vi "SVA 4MV6 T022 CCE.vi"(11 "SP":dbl(slide) scale=0.0..360.0) -> (3 "Posicion":cluster{dbl, dbl}(knob)={0.0, 349.0774854239136})   [LabVIEW 2020]
doc: "Ceballos Conde Emanuel 4MV6 Sistemas de visión artificial 2022/1\nEste VI realiza el control difuso de un SISTEMA SISO representado por un motor,el sisita tiene como entrada tiene la posición deseada y como salida un indicador de dos agujas donde la azul representa el valor solicitado y la roja el valor real"
uses:
  <vilib>/addons/Fuzzy Logic/TypeDefs/FL Defuzzification.ctl
  <vilib>/addons/Fuzzy Logic/TypeDefs/FL Antecedent Connective.ctl
  <vilib>/addons/Fuzzy Logic/TypeDefs/FL Consequent Implication.ctl
  <vilib>/addons/Fuzzy Logic/TypeDefs/FL Modifier.ctl
  <vilib>/addons/Fuzzy Logic/Membership/FL Create Membership Function (Triangle).vi
  <vilib>/addons/Fuzzy Logic/Membership/FL Create Membership Function (Trapezoid).vi
  <vilib>/addons/Fuzzy Logic/FL Fuzzy Controller (SISO).vi
  <vilib>/addons/Fuzzy Logic/NI_Fuzzy_Logic_API.lvlib
panel:
  in  "stop":bool
  # "Ceballos Conde Emanuel\n4MV6\nSistemas de visión artificial\n2022/1"
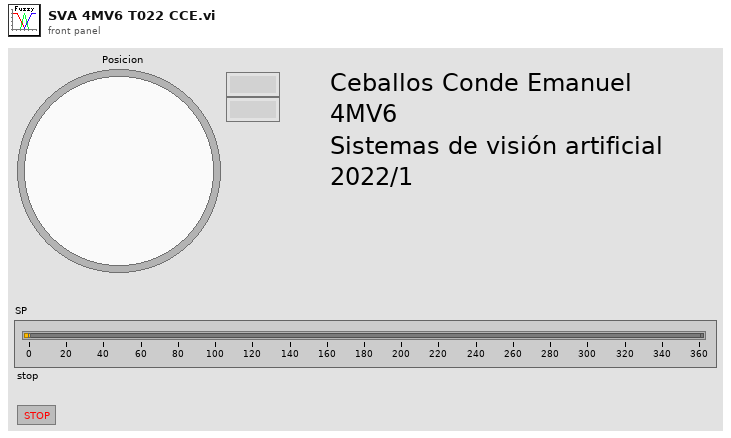
[diagram p1: front panel]
types:
  T1 = typedef "NI_Fuzzy_Logic_API.lvlib/FL Defuzzification.ctl" = u16
  T2 = typedef "NI_Fuzzy_Logic_API.lvlib/FL Membership Function.ctl" = cluster{"name":string, "shape":T3, "points":dbl[], "color":u32, "user-defined shape index":i32}
  T3 = typedef "NI_Fuzzy_Logic_API.lvlib/FL Membership Function Shape.ctl" = u16
  T4 = typedef "NI_Fuzzy_Logic_API.lvlib/FL Modifier.ctl" = u16
  T5 = typedef "NI_Fuzzy_Logic_API.lvlib/FL Consequent Implication.ctl" = u16
  T6 = typedef "NI_Fuzzy_Logic_API.lvlib/FL Antecedent Connective.ctl" = u16
  T7 = typedef "NI_Fuzzy_Logic_API.lvlib/FL Antecedent.ctl" = cluster{"Var Index":i32, "MF Index":i32, "Cond":T4}
  T8 = typedef "NI_Fuzzy_Logic_API.lvlib/FL Consequent.ctl" = cluster{"Var Index":i32, "MF Index":i32, "Cond":T4}
  T9 = typedef "NI_Fuzzy_Logic_API.lvlib/FL Rule.ctl" = cluster{"antecedents":T7[], "antecedent connective":T6, "consequents":T8[], "consequent implication":T5, "degree of support":dbl}
  T10 = typedef "NI_Fuzzy_Logic_API.lvlib/FL Variable.ctl" = cluster{"name":string, "range":dbl[], "MFs":T2[]}
  T11 = typedef "NI_Fuzzy_Logic_API.lvlib/FL System.ctl" = cluster{"input variables":T10[], "output variables":T10[], "rules":T9[], "defuzzification method":T1, "description":string, "user MF interpolating polynomials":T12[]}
  T12 = typedef "NI_Fuzzy_Logic_API.lvlib/FL Interpolating polynomials.ctl" = cluster{"X":dbl[], "Y":dbl[], "Y(x) coeff":dbl[][], "X(y) coeff":dbl[][], "Area(y) coeff":dbl[][], "coa_x(y) coeff":dbl[][]}
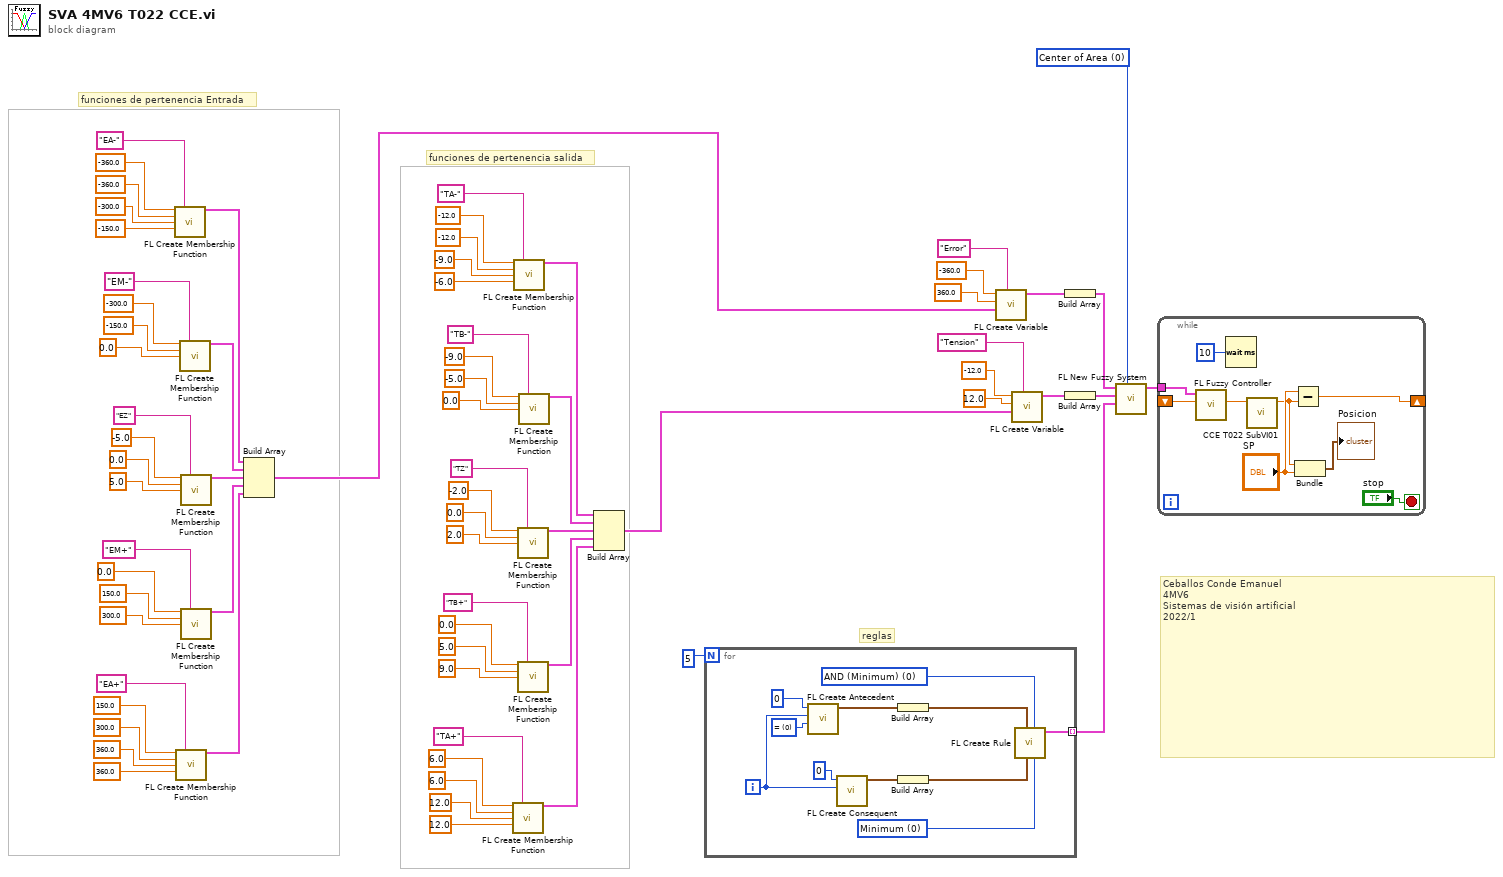
[diagram p0: block diagram]
diagram:
  w4 = T1 0 items=["Center of Area", "Modified Center of Area", "Center of Sums", "Center of Maximum", "Mean of Maximum"] ("defuzzification method")
  # "reglas"
  # "funciones de pertenencia salida"
  # "funciones de pertenencia Entrada"
  # "Ceballos Conde Emanuel\n4MV6\nSistemas de visión artificial\n2022/1"
  n1 = call-poly <vilib>:"FL Create Membership Function.vi"("left base"=-360.0, "name"="EA-", "left top"=-360.0 ("top"), "right top"=-300.0 ("right base"), "right base"=-150.0) -> ("membership function"=w63:T2)  [unwired: 9 in, 1 out]
  n2 = call-poly <vilib>:"FL Create Membership Function.vi"("left base"=150.0, "name"="EA+", "left top"=300.0 ("top"), "right top"=360.0 ("right base"), "right base"=360.0) -> ("membership function"=w42:T2)  [unwired: 9 in, 1 out]
  n3 = call-poly <vilib>:"FL Create Membership Function.vi"("left base"=-300.0, "name"="EM-", "top"=-150.0, "right base"=0.0) -> ("membership function"=w57:T2)  [unwired: 10 in, 1 out]
  n4 = call-poly <vilib>:"FL Create Membership Function.vi"("left base"=-5.0, "name"="EZ", "top"=0.0, "right base"=5.0) -> ("membership function"=w52:T2)  [unwired: 10 in, 1 out]
  n5 = call-poly <vilib>:"FL Create Membership Function.vi"("left base"=0.0, "name"="EM+", "top"=150.0, "right base"=300.0) -> ("membership function"=w47:T2)  [unwired: 10 in, 1 out]
  n6 = Build Array(w63, w57, w52, w47, w42) -> (w62:T2[])
  n7 = call-poly <vilib>:"FL Create Membership Function.vi"("left base"=6.0, "name"="TA+", "left top"=6.0 ("top"), "right top"=12.0 ("right base"), "right base"=12.0) -> ("membership function"=w9:T2)  [unwired: 9 in, 1 out]
  n8 = call-poly <vilib>:"FL Create Membership Function.vi"("left base"=-12.0, "name"="TA-", "left top"=-12.0 ("top"), "right top"=-9.0 ("right base"), "right base"=-6.0) -> ("membership function"=w30:T2)  [unwired: 9 in, 1 out]
  n9 = call-poly <vilib>:"FL Create Membership Function.vi"("left base"=-2.0, "name"="TZ", "top"=0.0, "right base"=2.0) -> ("membership function"=w19:T2)  [unwired: 10 in, 1 out]
  n10 = call-poly <vilib>:"FL Create Membership Function.vi"("left base"=0.0, "name"="TB+", "top"=5.0, "right base"=9.0) -> ("membership function"=w14:T2)  [unwired: 10 in, 1 out]
  n11 = call-poly <vilib>:"FL Create Membership Function.vi"("left base"=-9.0, "name"="TB-", "top"=-5.0, "right base"=0.0) -> ("membership function"=w24:T2)  [unwired: 10 in, 1 out]
  n12 = Build Array(w30, w24, w19, w14, w9) -> (w29:T2[])
  n13 = for {
    N: 5 -> [_]
    tunnel: [w71] -> w2 mode=indexing
    i -> [w74]
    w77 = T4 0 items=["=", "!="] ("condition")
    w80 = T5 0 items=["Minimum", "Product"] ("consequent implication")
    w81 = T6 0 items=["AND (Minimum)", "AND (Product)", "OR (Maximum)", "OR (Probabilistic)"] ("antecedent connective")
    n14 = call <vilib>:"FL Create Antecedent.vi"("condition"=w77, "membership function index"=w74, "variable index"=0) -> ("antecedent"=w79:T7)  [unwired: 7 in, 1 out]
    n15 = call <vilib>:"FL Create Consequent.vi"("membership function index"=w74, "variable index"=0) -> ("consequent"=w78:T8)  [unwired: 8 in, 1 out]
    n16 = Build Array(w79) -> (w73:T7[])
    n17 = Build Array(w78) -> (w72:T8[])
    n18 = call <vilib>:"FL Create Rule.vi"("consequent implication"=w80, "antecedent connective"=w81, "consequents"=w72, "antecedents"=w73) -> ("rule"=w71:T9)  [unwired: 6 in, 1 out]
  }
  n19 = call <vilib>:"FL Create Variable.vi"("name"="Error", "membership functions"=w62, "maximum"=360.0, "minimum"=-360.0) -> ("variable"=w40:T10)  [unwired: 6 in, 1 out]
  n20 = call <vilib>:"FL Create Variable.vi"("name"="Tension", "membership functions"=w29, "maximum"=12.0, "minimum"=-12.0) -> ("variable"=w7:T10)  [unwired: 6 in, 1 out]
  n21 = Build Array(w40) -> (w39:T10[])
  n22 = Build Array(w7) -> (w5:T10[])
  n23 = call <vilib>:"FL New Fuzzy System.vi"("defuzzification method"=w4, "rules"=w2, "output variables"=w5, "input variables"=w39) -> ("fuzzy system out"=w1:T11)  [unwired: 6 in, 1 out]
  n24 = while {
    shift-right: [w88] -> _
    shift-left: _ -> [w86]
    tunnel: w1 -> [w87]
    stop <- "stop" stop-if-true
    n25 = call-poly <vilib>:"FL Fuzzy Controller.vi"("input value"=w86, "fuzzy system in"=w87) -> ("output value"=w85:dbl)  [unwired: 5 in, 4 out]
    n26 = Wait (ms)(milliseconds to wait=u32 10) -> ()  [unwired: 1 out]
    n27 = call "CCE T022 SubVI01.vi"("Tensión"=w85) -> ("Posicion"=w82:dbl)  [unwired: 10 in]
    n28 = Subtract(x="SP", y=w82) -> (x-y=w88:dbl)
    n29 = Bundle("Posicion"=w82, "SP"="SP") -> (→"Posicion":cluster{"Posicion":dbl, "SP":dbl})  [unwired: 1 in]
  }
